vi "GetStatusLine.vi"(3 "Status":T1[](array[typedef])) -> (0 "all good?":bool, 1 "Status":string)   [LabVIEW 2012]
uses:
  _ROSDefinition.vi
  MyState.ctl
panel:
  out "h(x)":i32[](array[numeric])
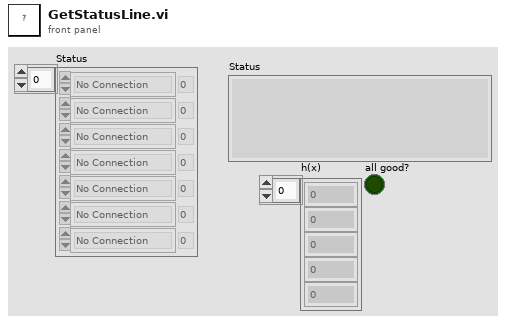
[diagram p1: front panel]
types:
  T1 = typedef "MyState.ctl" = enum16{"No Connection", "Registered", "Connected", "Close"}
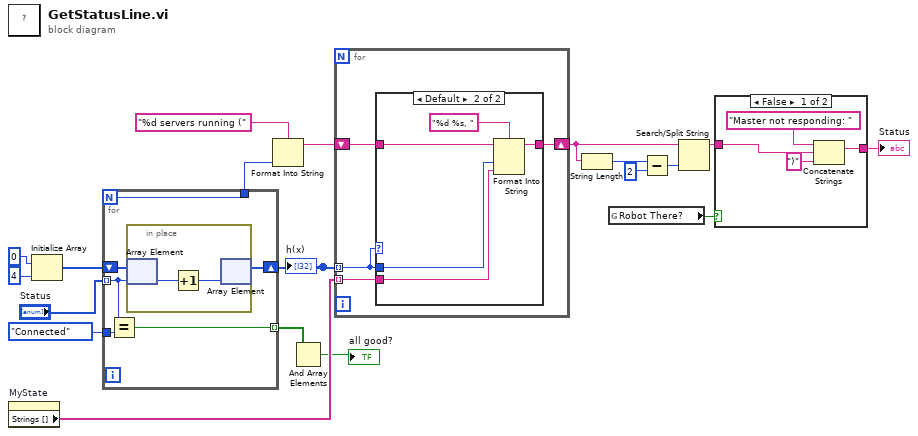
[diagram p0: block diagram]
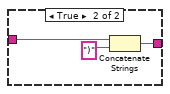
[diagram p2: hidden frame]
diagram:
  n1 = property on="MyState" class="Enum (strict)"() -> ("Strings []"=w19:string[])  [unwired: 2 in, 2 out]
  n2 = Initialize Array(u8 0 ("element"), 4 ("dimension size")) -> (w15:u8[])
  n3 = for {
    N -> [w23]
    shift-right: [w24] -> w11
    shift-left: w15 -> [w25]
    tunnel: "Status" -> [w21] mode=indexing
    tunnel: [w23] -> w5
    tunnel: MyState."Connected" ("MyState") -> [w22]
    tunnel: [w20] -> w2 mode=indexing
    n4 = Equal?(x=w21, y=w22) -> (x = y?=w20:bool)
    n5 = in-place {
      n6 = in-place-array #1(w25, w21) -> (w27:u8)
      n7 = Increment(x=w27) -> (x+1=w26:u8)
      n8 = in-place-array #1(w26) -> (w24:u8[])  [unwired: 1 out]
    }
  }
  "h(x)" <- w11
  n9 = Format Into String(format string="%d servers running (" ("regular expression"), w5) -> (resulting string=w16:string)  [unwired: 2 in, 1 out]
  n10 = And Array Elements(Boolean array=w2) -> (logical AND=→"all good?":bool)
  n11 = for {
    shift-right: [w30] -> w9
    shift-left: w16 -> [w31]
    tunnel: w19 -> [w29] mode=indexing
    tunnel: w11 -> [w28] mode=indexing
    n12 = case shown="Default" w28 {
      tunnel: w31 -> [w32 w37]
      tunnel: [w32 w36] -> w30
      tunnel: w29 -> [_ w34]
      tunnel: w28 -> [_ w33]
      frame 0 {
      }
      frame Default {
        n13 = Format Into String(format string="%d %s, ", initial string=w37, w33, w34) -> (resulting string=w36:string)  [unwired: 1 in, 1 out]
      }
    }
  }
  n14 = String Length(string=w9) -> (length=w8:i32)
  n15 = global read "_ROSDefinition.vi" "Robot There?"() -> (w4:bool)
  n16 = Subtract(x=w8, y=2) -> (x-y=w6:i32)
  n17 = Search/Split String(string=w9, offset (0)=w6) -> (substring before match=w10:string)  [unwired: 1 in, 2 out]
  n18 = case shown="False" w4 {
    tunnel: [w39 w43] -> w18
    tunnel: w10 -> [w40 w42]
    frame False {
      n19 = Concatenate Strings("Master not responding: ", w40, ")" ("string")) -> (w39:string)
    }
    frame True {
      n20 = Concatenate Strings(w42, ")" ("string")) -> (w43:string)
    }
  }
  "Status" <- w18
